vi "SizeOrderedMorphology.vi"(2 "Report Size Limit":i32=3, 3 "Image Dst Out":T2) -> (0 "Particles":T1(array[cluster]), 1 "Particles":i32)   [LabVIEW 2013]
uses:
  <vilib>/vision/Image Controls.llb/IMAQ Image.ctl
  <vilib>/vision/NI_Vision_Development_Module.lvlib
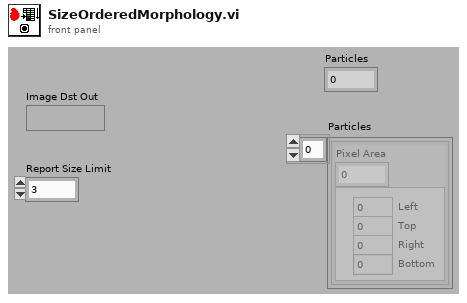
[diagram p1: front panel]
types:
  T1 = cluster{"Pixel Area":dbl, "Rectangle":cluster{"Left":i32, "Top":i32, "Right":i32, "Bottom":i32}}[]
  T2 = typedef "IMAQ Image.ctl" = refnum<image>
  T3 = typedef "Particle Parameters" = i32
  T4 = cluster{"Numeric":dbl, "Numeric":dbl, "Numeric":dbl, "Numeric":dbl}
  T5 = cluster{"Numeric":dbl, cluster{"Numeric":dbl, "Numeric":dbl, "Numeric":dbl, "Numeric":dbl}}
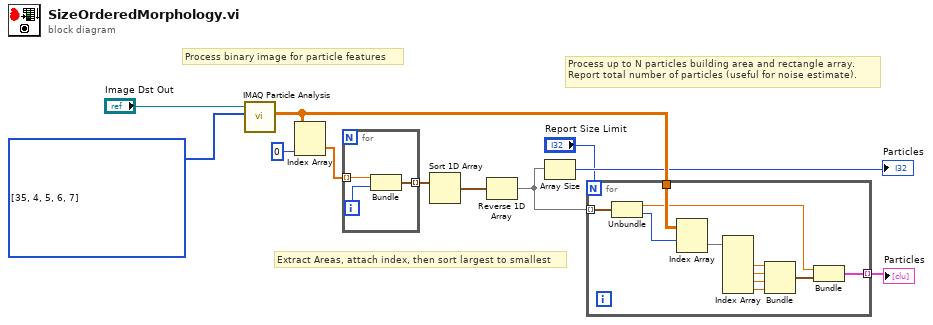
[diagram p0: block diagram]
diagram:
  w6 = T3[] [35, 4, 5, 6, 7] items=["Center of Mass X", "Center of Mass Y", "First Pixel X", "First Pixel Y", "Bounding Rect Left", "Bounding Rect Top", "Bounding Rect Right", "Bounding Rect Bottom", "Max Feret Diameter Start X", "Max Feret Diameter Start Y", "Max Feret Diameter End X", "Max Feret Diameter End Y", "Max Horiz. Segment Length Left", "Max Horiz. Segment Length Right", "Max Horiz. Segment Length Row", "-", "Bounding Rect Width", "Bounding Rect Height", "Bounding Rect Diagonal", "Perimeter", "Convex Hull Perimeter", "Holes' Perimeter", "Max Feret Diameter", "Equivalent Ellipse Major Axis", "Equivalent Ellipse Minor Axis", "Equivalent Ellipse Minor Axis (Feret)", "Equivalent Rect Long Side", "Equivalent Rect Short Side", "Equivalent Rect Diagonal", "Equivalent Rect Short Side (Feret)", "Average Horiz. Segment Length", "Average Vert. Segment Length", "Hydraulic Radius", "Waddel Disk Diameter", "-", "Area", "Holes' Area", "Particle & Holes' Area", "Convex Hull Area", "Image Area", "-", "Number of Holes", "Number of Horiz. Segments", "Number of Vert. Segments", "-", "Orientation", "Max Feret Diameter Orientation", "-", "% Area/Image Area", "% Area/(Particle & Holes' Area)", "Ratio of Equivalent Ellipse Axes", "Ratio of Equivalent Rect Sides", "-", "Elongation Factor", "Compactness Factor", "Heywood Circularity Factor", "Type Factor", "-", "Sum X", "Sum Y", "Sum XX", "Sum XY", "Sum YY", "Sum XXX", "Sum XXY", "Sum XYY", "Sum YYY", "-", "Moment of Inertia XX", "Moment of Inertia XY", "Moment of Inertia YY", "Moment of Inertia XXX", "Moment of Inertia XXY", "Moment of Inertia XYY", "Moment of Inertia YYY", "Norm. Moment of Inertia XX", "Norm. Moment of Inertia XY", "Norm. Moment of Inertia YY", "Norm. Moment of Inertia XXX", "Norm. Moment of Inertia XXY", "Norm. Moment of Inertia XYY", "Norm. Moment of Inertia YYY", "Hu Moment 1", "Hu Moment 2", "Hu Moment 3", "Hu Moment 4", "Hu Moment 5", "Hu Moment 6", "Hu Moment 7"] ("Pixel Measurements")
  # "Process up to N particles building area and rectangle array.\nReport total number of particles (useful for noise estimate)."
  # "Process binary image for particle features"
  # "Extract Areas, attach index, then sort largest to smallest"
  n1 = call "IMAQ Particle Analysis"("Pixel Measurements"=w6, "Image"="Image Dst Out") -> ("Particle Measurements (Pixels)"=w5:dbl[][])  [unwired: 3 in, 6 out]
  n2 = Index Array(array=w5, index (col)=0 ("disabled index (col)")) -> (element=w8:dbl[])  [unwired: 1 in]
  n3 = for {
    tunnel: w8 -> [w14] mode=indexing
    tunnel: [w13] -> w9 mode=indexing
    i -> [w12]
    n4 = Bundle("Numeric"=w14, w12) -> (w13:cluster{"Numeric":dbl, i32})  [unwired: 1 out]
  }
  n5 = Sort 1D Array(array=w9) -> (sorted array=w10:cluster{"Numeric":dbl, i32}[])
  n6 = Reverse 1D Array(array=w10) -> (reversed array=w3:cluster{"Numeric":dbl, i32}[])
  n7 = Array Size(array=w3) -> (size(s)=→"Particles":i32)
  n8 = for {
    N: "Report Size Limit" -> [_]
    tunnel: w5 -> [w20]
    tunnel: w3 -> [w18] mode=indexing
    tunnel: [w17] -> w2 mode=indexing
    n9 = Unbundle(w18) -> ("Numeric"=w16:dbl, w25:i32)
    n10 = Index Array(array=w20, index (row)=w25) -> (element=w19:dbl[])  [unwired: 1 in]
    n11 = Index Array(array=w19) -> (element #2=w24:dbl, element #3=w23:dbl, element #4=w22:dbl, element #5=w21:dbl)  [unwired: 5 in, 1 out]
    n12 = Bundle("Numeric"=w24, "Numeric"=w23, "Numeric"=w22, "Numeric"=w21) -> (w15:T4)  [unwired: 1 out]
    n13 = Bundle("Numeric"=w16, w15) -> (w17:T5)  [unwired: 1 out]
  }
  "Particles" <- w2
